vi "CFTS-Read Options.vi"(8 "error in (no error)":errorcluster) -> (0 "error out":errorcluster, 3 "CFTS Options":T1)   [LabVIEW 2020]
uses:
  CFTS-Options.ctl
panel:
  in  "CFTS Default Options":T1
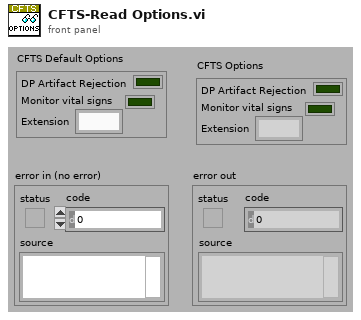
[diagram p1: front panel]
types:
  T1 = typedef "CFTS-Options.ctl" = cluster{"DP Artifact Rejection":bool, "Monitor vital signs ":bool, "Extension":string}
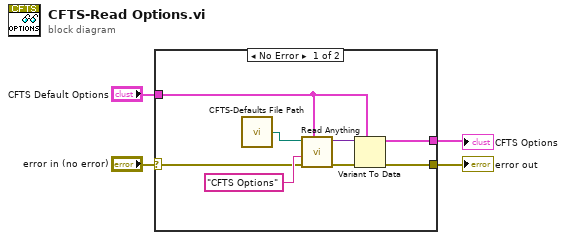
[diagram p0: block diagram]
diagram:
  n1 = case shown="No Error" "error in (no error)" {
    selector: "error in (no error)" -> [w11 w14]
    tunnel: [w7 w14] -> w4
    tunnel: "CFTS Default Options" -> [w6 w13]
    tunnel: [w8 w13] -> w1
    frame No Error {
      n2 = call "CFTS-Defaults File Path.vi"() -> ("Path"=w5:path)  [unwired: 1 in]
      n3 = call "Read Anything.vi"("Type of Anything"=w6, "Error In"=w11, "Section Name (Name of \"Type of Anything\")"="CFTS Options" ("Section Name (Name of \"Type of Anything\")"), "Path (dialog)"=w5) -> ("Error Out"=w10:errorcluster, "Anything"=w9:variant)  [unwired: 5 in, 1 out]
      n4 = Variant To Data(error in=w10, type=w6, Variant=w9) -> (data=w8:T1, error out=w7:errorcluster)
    }
    frame Error {
    }
  }
  "error out" <- w4
  "CFTS Options" <- w1
